vi "Oscillator.vi"(1 "OscillatorInfo":T2={"frequency"=10.0, "amplitude"=1.0, "sample rate"=0, "waveform type"=enum."Sine"}) -> (0 "output sample":dbl)   [LabVIEW 2016]
uses:
  Oscillator/WaveformType.ctl
  <vilib>/measure/NI_MABase.lvlib
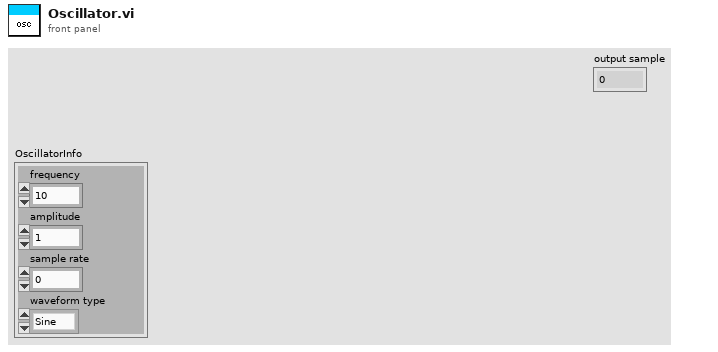
[diagram p1: front panel]
types:
  T1 = typedef "WaveformType.ctl" = enum16{"Sine", "Triangle", "Square", "Sawtooth"}
  T2 = cluster{"frequency":dbl, "amplitude":dbl, "sample rate":i32, "waveform type":T1}
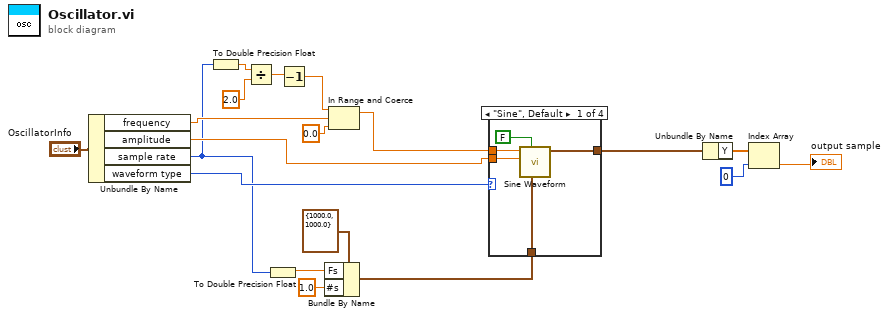
[diagram p0: block diagram]
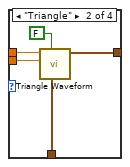
[diagram p2: hidden frame]
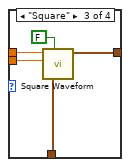
[diagram p3: hidden frame]
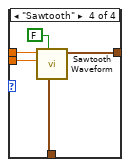
[diagram p4: hidden frame]
diagram:
  n1 = Unbundle By Name("OscillatorInfo") -> ("frequency"=w7:dbl, "amplitude"=w12:dbl, "sample rate"=w5:i32, "waveform type"=w13:T1)
  n2 = To Double Precision Float(number=w5) -> (double precision float=w4:dbl)
  n3 = Divide(x=w4, y=2.0) -> (x/y=w2:dbl)
  n4 = To Double Precision Float(number=w5) -> (double precision float=w18:dbl)
  n5 = Decrement(x=w2) -> (x-1=w1:dbl)
  n6 = Bundle By Name(cluster=cluster{"Fs":dbl, "#s":dbl} {"Fs"=1000.0, "#s"=1000.0} ("sampling info"), "Fs"=w18, "#s"=1.0) -> (w16:cluster{"Fs":dbl, "#s":dbl})
  n7 = In Range and Coerce(upper limit=w1, x=w7, lower limit=0.0) -> (coerced(x)=w8:dbl)  [unwired: 1 out]
  n8 = case shown="\"Sine\", Default" w13 {
    tunnel: w8 -> [w24 w29 w34 w39]
    tunnel: w12 -> [w23 w28 w33 w38]
    tunnel: w16 -> [w22 w26 w31 w36]
    tunnel: [w21 w27 w32 w37] -> w15
    frame "Sine", Default {
      n9 = call <vilib>:"Sine Waveform.vi"("sampling info"=w22, "reset signal"=FALSE, "amplitude"=w23, "frequency"=w24) -> ("signal out"=w21:waveform(dbl))  [unwired: 6 in, 1 out]
    }
    frame "Triangle" {
      n10 = call <vilib>:"Triangle Waveform.vi"("sampling info"=w26, "reset signal"=FALSE, "amplitude"=w28, "frequency"=w29) -> ("signal out"=w27:waveform(dbl))  [unwired: 6 in, 1 out]
    }
    frame "Square" {
      n11 = call <vilib>:"Square Waveform.vi"("sampling info"=w31, "reset signal"=FALSE, "amplitude"=w33, "frequency"=w34) -> ("signal out"=w32:waveform(dbl))  [unwired: 6 in, 1 out]
    }
    frame "Sawtooth" {
      n12 = call <vilib>:"Sawtooth Waveform.vi"("sampling info"=w36, "reset signal"=FALSE, "amplitude"=w38, "frequency"=w39) -> ("signal out"=w37:waveform(dbl))  [unwired: 6 in, 1 out]
    }
  }
  n13 = Unbundle By Name(w15) -> ("Y"=w11:dbl[])
  n14 = Index Array(array=w11, index=0) -> (element=→"output sample":dbl)
